vi "TS Acq Start.vi"(8 "error in":errorcluster, 11 "HTS Test Stand in":refnum<class "HTS Test Stand.lvclass">) -> (0 "error out":errorcluster, 3 "HTS Test Stand out":refnum<class "HTS Test Stand.lvclass">)   [LabVIEW 2019, in "Test Stands.lvlib" / "HTS Test Stand.lvclass"]
uses:
  HTS Test Stand.lvclass
  DAC/HTS/Vacum Valve/DAC Vacum Valve.lvclass
  Generic Test Stand/Generic Test Stand.lvclass/Generic Test Stand.ctl
  DAC/HTS/Vacum Valve/DAC Vacum Valve.lvclass/DAC Vacum Valve.ctl
  DAC/DAC.lvclass
  C:/Users/wg/Documents/LV_Projects/test-stand/App/DAC/DAC.lvclass
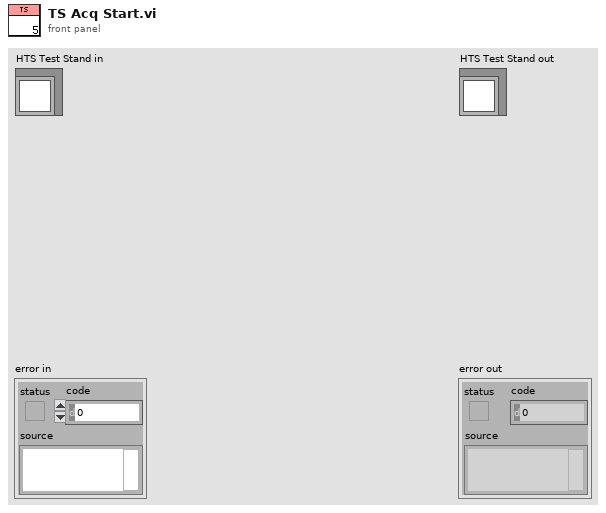
[diagram p1: front panel]
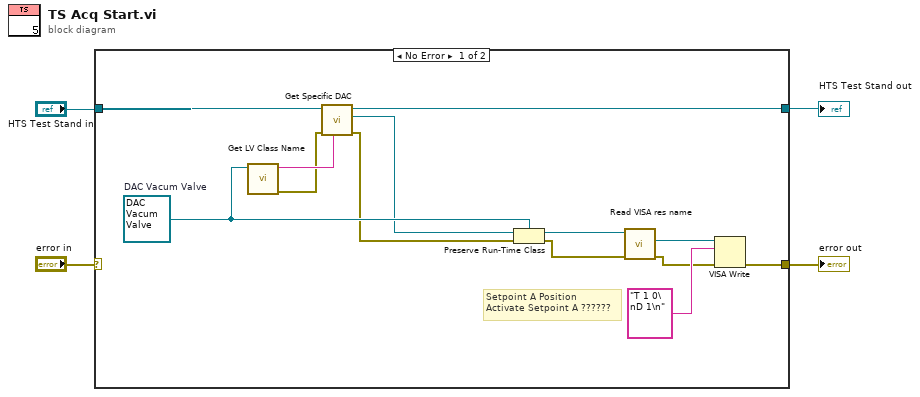
[diagram p0: block diagram]
diagram:
  n1 = case shown="No Error" "error in" {
    selector: "error in" -> [_ w19]
    tunnel: [w14 w19] -> w1
    tunnel: [w9 w18] -> w3
    tunnel: "HTS Test Stand in" -> [w11 w18]
    frame No Error {
      w10 = refnum<class "DAC Vacum Valve.lvclass"> refnum  # DAC Vacum Valve
      # "Setpoint A Position\nActivate Setpoint A ??????"
      n2 = call <vilib>:"Get LV Class Name.vi"("object"=w10) -> ("error out"=w12:errorcluster, "class name"=w13:string)  [unwired: 9 in]
      n3 = call-dynamic "Get Specific DAC.vi"("DAC Class Name"=w13, "error in"=w12, "Generic Test Stand in"=w11) -> ("error out"=w7:errorcluster, "DAC"=w8:refnum<class "DAC.lvclass">, "Generic Test Stand out"=w9:refnum<class "HTS Test Stand.lvclass">)  [unwired: 6 in]
      n4 = Preserve Run-Time Class(object in=w8, error in=w7, 2:w10) -> (object out=w17:refnum<class "DAC Vacum Valve.lvclass">, error out=w6:errorcluster)
      n5 = call "Read VISA res name.vi"("error in (no error)"=w6, "DAC Vacum Valve in"=w17) -> ("error out"=w5:errorcluster, "VISA res name"=w16:refnum<visa-resource-name>)  [unwired: 7 in, 1 out]
      n6 = VISA Write(VISA resource name=w16, write buffer="T 1 0\nD 1\n", error in (no error)=w5) -> (error out=w14:errorcluster)  [unwired: 2 out]
    }
    frame Error {
    }
  }
  "error out" <- w1
  "HTS Test Stand out" <- w3
